vi "s-3 yazılan değere iki ekleyip diziye 5 kere yazan program 2018 19.vi"() -> ()   [LabVIEW 2014]
panel:
  out "Array":dbl[](array[numeric])
  in  "Numeric":dbl
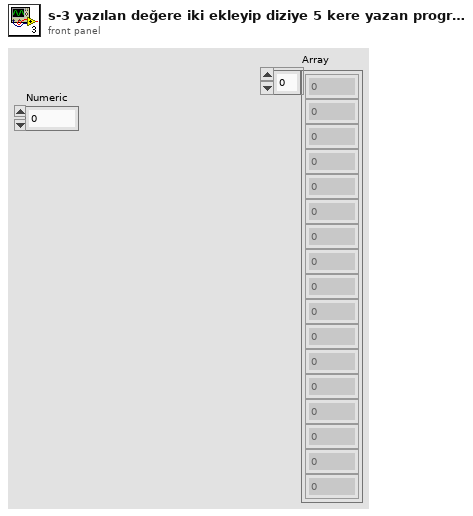
[diagram p1: front panel]
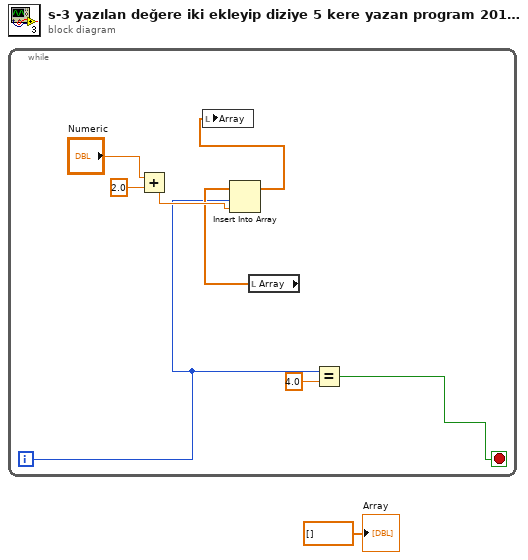
[diagram p0: block diagram]
diagram:
  n1 = while {
    i -> [w2]
    stop <- w3 stop-if-true
    n2 = Add(x="Numeric", y=2.0) -> (x+y=w7:dbl)
    n3 = local read "Array"() -> (w5:dbl[])
    n4 = Insert Into Array(array=w5, index=w2, new element=w7) -> (w6:dbl[])
    n5 = local write "Array"(w6) -> ()
    n6 = Equal?(x=w2, y=4.0) -> (x = y?=w3:bool)
  }
  "Array" <- dbl[] [] ("Array")
